vi "Configure Trace Type.vi"(6 "Enable Trace Display (F: Disable)":bool, 7 "Enable Trace Update (F: Disable)":bool, 8 "error in (no error)":errorcluster, 9 "Trace Type (0: Clear Write)":i32(ring) items=["Clear Write", "Average", "Maximum Hold", "Minimum Hold"], 10 "Trace Name (1: Trace 1)":i32(ring)=1 items=["Trace 1"=1, "Trace 2"=2, "Trace 3"=3, "Trace 4"=4, "Trace 5"=5, "Trace 6"=6], 11 "VISA resource name":refnum<visa-resource-name>) -> (0 "error out":errorcluster, 3 "VISA resource name out":refnum<visa-resource-name>)   [LabVIEW 2014, in "Agilent MXA Series.lvlib"]
doc: "Configures the type of trace to acquire.\n\n<B>Note:</B>\nYou can use this vi only under Swept SA measurement type."
uses:
  Agilent MXA Series.lvlib
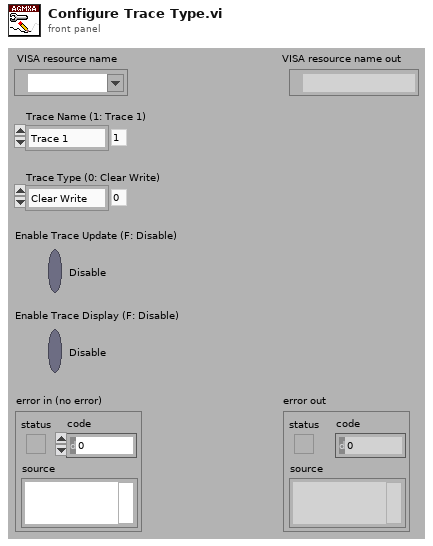
[diagram p1: front panel]
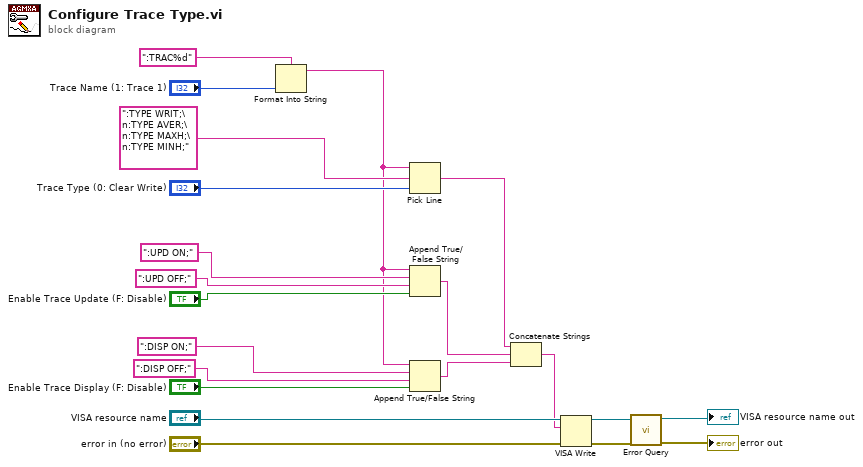
[diagram p0: block diagram]
diagram:
  n1 = Format Into String(format string=":TRAC%d" ("string (\"\")"), "Trace Name (1: Trace 1)") -> (resulting string=w1:string)  [unwired: 2 in, 1 out]
  n2 = Pick Line(string ("")=w1, multi-line string=":TYPE WRIT;\n:TYPE AVER;\n:TYPE MAXH;\n:TYPE MINH;", line index="Trace Type (0: Clear Write)") -> (output string=w5:string)
  n3 = Append True/False String(1:"Enable Trace Update (F: Disable)", 2:":UPD OFF;" ("string"), 3:":UPD ON;" ("string"), 4:w1) -> (0:w4:string)
  n4 = Append True/False String(1:"Enable Trace Display (F: Disable)", 2:":DISP OFF;" ("string"), 3:":DISP ON;" ("string"), 4:w1) -> (0:w3:string)
  n5 = Concatenate Strings(w5, w4, w3) -> (w2:string)
  n6 = VISA Write(VISA resource name="VISA resource name", write buffer=w2, error in (no error)="error in (no error)") -> (VISA resource name out=w15:refnum<visa-resource-name>, error out=w14:errorcluster)  [unwired: 1 out]
  n7 = call "Error Query.vi"("error in (no error)"=w14, "VISA resource name"=w15) -> ("error out"=→"error out":errorcluster, "VISA resource name out"=→"VISA resource name out":refnum<visa-resource-name>)  [unwired: 6 in, 2 out]
